vi "Agilent 3352X Series Standard Waveform2.vi"() -> ()   [LabVIEW 2015]
doc: "This example shows how to generate a standard waveform."
uses:
  Agilent 3352X Series.lvlib
panel:
  in  "stop":bool
  in  "DC Offset (0 V)":dbl=0.65
  in  "Waveform Function (0: Sine)":u16(ring)=5 items=["Sine"=0, "Square"=1, "Ramp"=2, "Noise"=3, "DC"=4, "Triangle"=5, "Pulse"=6, "Sinc"=11, "D-Lorentz"=12, "Gaussian"=13, "Expo Fall"=14, "Expo Rise"=15, "Haversine"=16]
  in  "Frequency/Sample Rate/Bandwidth (1000 Hz)":dbl=537.0
  in  "Amplitude (0.1 Vpp)":dbl=1.2
  in  "VISA resource name":refnum<visa-resource-name>="USB0::0x0957::0x5707::MY53801762::INSTR"
  # "(c) 2011-2015 National Instruments.  ALL RIGHTS RESERVED."
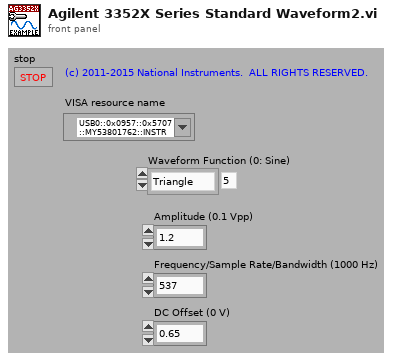
[diagram p1: front panel]
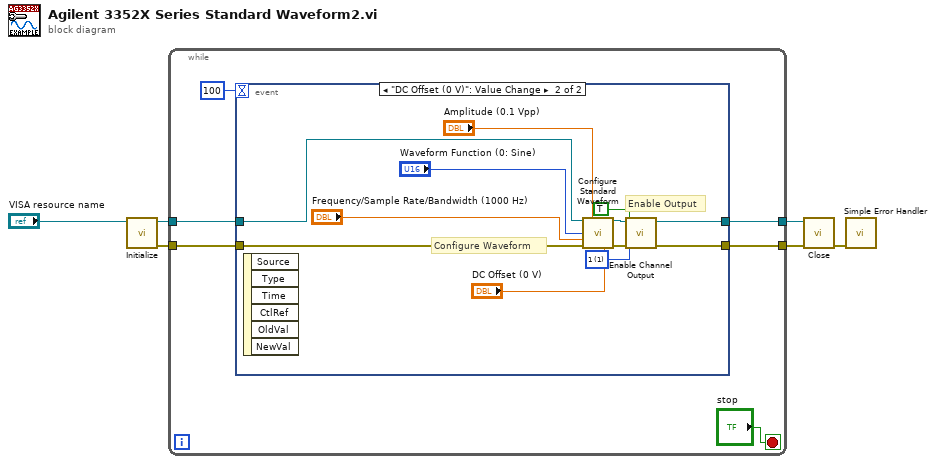
[diagram p0: block diagram]
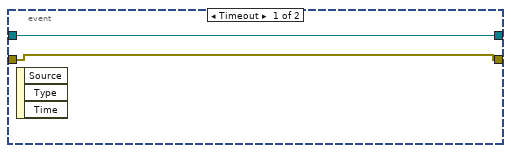
[diagram p2: hidden frame]
diagram:
  n1 = call "Initialize.vi"("VISA resource name"="VISA resource name") -> ("error out"=w2:errorcluster, "VISA resource name out"=w1:refnum<visa-resource-name>)  [unwired: 4 in, 5 out]
  n2 = while {
    tunnel: w1 -> [w9]
    tunnel: [w12] -> w4
    tunnel: w2 -> [w10]
    tunnel: [w11] -> w3
    stop <- "stop" stop-if-true
    n3 = event shown="[1] \"DC Offset (0 V)\": Value Change" {
      selector: _ -> [_ _]
      dyn-events: _ -> [_ _]
      timeout: 100 -> [_ _]
      tunnel: [w14 w19] -> w12
      tunnel: [w13 w20] -> w11
      tunnel: w10 -> [w13 w18]
      tunnel: w9 -> [w14 w17]
      event Timeout {
        n4 = event-data() -> ()  [unwired: 1 in, 3 out]
      }
      event "DC Offset (0 V)": Value Change {
        w15 = u16 1 items=["1"=1, "2"=2] ("Channel (1: 1)")
        # "Enable Output"
        # "Configure Waveform"
        n5 = event-data() -> ()  [unwired: 1 in, 6 out]
        n6 = call "Configure Standard Waveform.vi"("VISA resource name"=w17, "Amplitude (0.1 Vpp)"="Amplitude (0.1 Vpp)", "Waveform Function (0: Sine)"="Waveform Function (0: Sine)", "Frequency/Sample Rate/Bandwidth (1000 Hz)"="Frequency/Sample Rate/Bandwidth (1000 Hz)", "error in (no error)"=w18, "DC Offset (0 V)"="DC Offset (0 V)") -> ("VISA resource name out"=w26:refnum<visa-resource-name>, "error out"=w25:errorcluster)  [unwired: 4 in, 4 out]
        n7 = call "Enable Channel Output.vi"("error in (no error)"=w25, "Channel (1: 1)"=w15, "Enable Output (T: Enable)"=TRUE, "VISA resource name"=w26) -> ("error out"=w20:errorcluster, "VISA resource name out"=w19:refnum<visa-resource-name>)  [unwired: 1 in, 5 out]
      }
    }
  }
  n8 = call "Close.vi"("error in (no error)"=w3, "VISA resource name"=w4) -> ("error out"=w5:errorcluster)  [unwired: 9 out]
  n9 = call <vilib>:"Simple Error Handler.vi"("error in (no error)"=w5) -> ()  [unwired: 1 in, 8 out]
